vi "Build Per Cycle CO CO2 Array.vi"(4 "Burner ON":bool, 6 "Start Analyzing Cycles at":u16=14, 7 "Conditions":T8, 8 "error in":errorcluster, 11 "PLC Data In":T1 {"PLC Data - LDO"."Timing"."Absolute Time" format="%<%H:%M:%S%3u>t"; "PLC Data - LDO"."Timing"."Display Time" format="%#.20f"; "PLC Data - LDO"."Timing"."Test Time Ref" format="%#.20f"; "PLC Data - LDO"."Timing"."Precondition Time Ref" format="%#.20f"; "PLC Data - LDO"."Timing"."First Call Time Ref" format="%#.20f"; "PLC Data - FVIR"."Timing"."Absolute Time" format="%<%H:%M:%S%3u>t"; "PLC Data - FVIR"."Timing"."Display Time" format="%#.20f"; "PLC Data - FVIR"."Timing"."Test Time Ref" format="%#.20f"; "PLC Data - FVIR"."Timing"."Precondition Time Ref" format="%#.20f"; "PLC Data - FVIR"."Timing"."First Call Time Ref" format="%#.20f"}) -> (0 "error out":errorcluster, 3 "PLC Data Out":T1 {"PLC Data - LDO"."Timing"."Absolute Time" format="%<%H:%M:%S%3u>t"; "PLC Data - LDO"."Timing"."Display Time" format="%#.20f"; "PLC Data - LDO"."Timing"."Test Time Ref" format="%#.20f"; "PLC Data - LDO"."Timing"."Precondition Time Ref" format="%#.20f"; "PLC Data - LDO"."Timing"."First Call Time Ref" format="%#.20f"; "PLC Data - FVIR"."Timing"."Absolute Time" format="%<%H:%M:%S%3u>t"; "PLC Data - FVIR"."Timing"."Display Time" format="%#.20f"; "PLC Data - FVIR"."Timing"."Test Time Ref" format="%#.20f"; "PLC Data - FVIR"."Timing"."Precondition Time Ref" format="%#.20f"; "PLC Data - FVIR"."Timing"."First Call Time Ref" format="%#.20f"})   [LabVIEW 2020]
uses:
  Terminate Condition ENUM.ctl
  Modbus/Modbus PLC Data All.ctl
  Modbus/Modbus FVIR Control.ctl
  Modbus/Modbus Timing.ctl
  <vilib>/Utility/miscctls.llb/LVDateTimeRec.ctl
  Modbus/Modbus LDO Control.ctl
  WritingDataFile/Data to Save.ctl
  Terminate Conditions Cluster.ctl
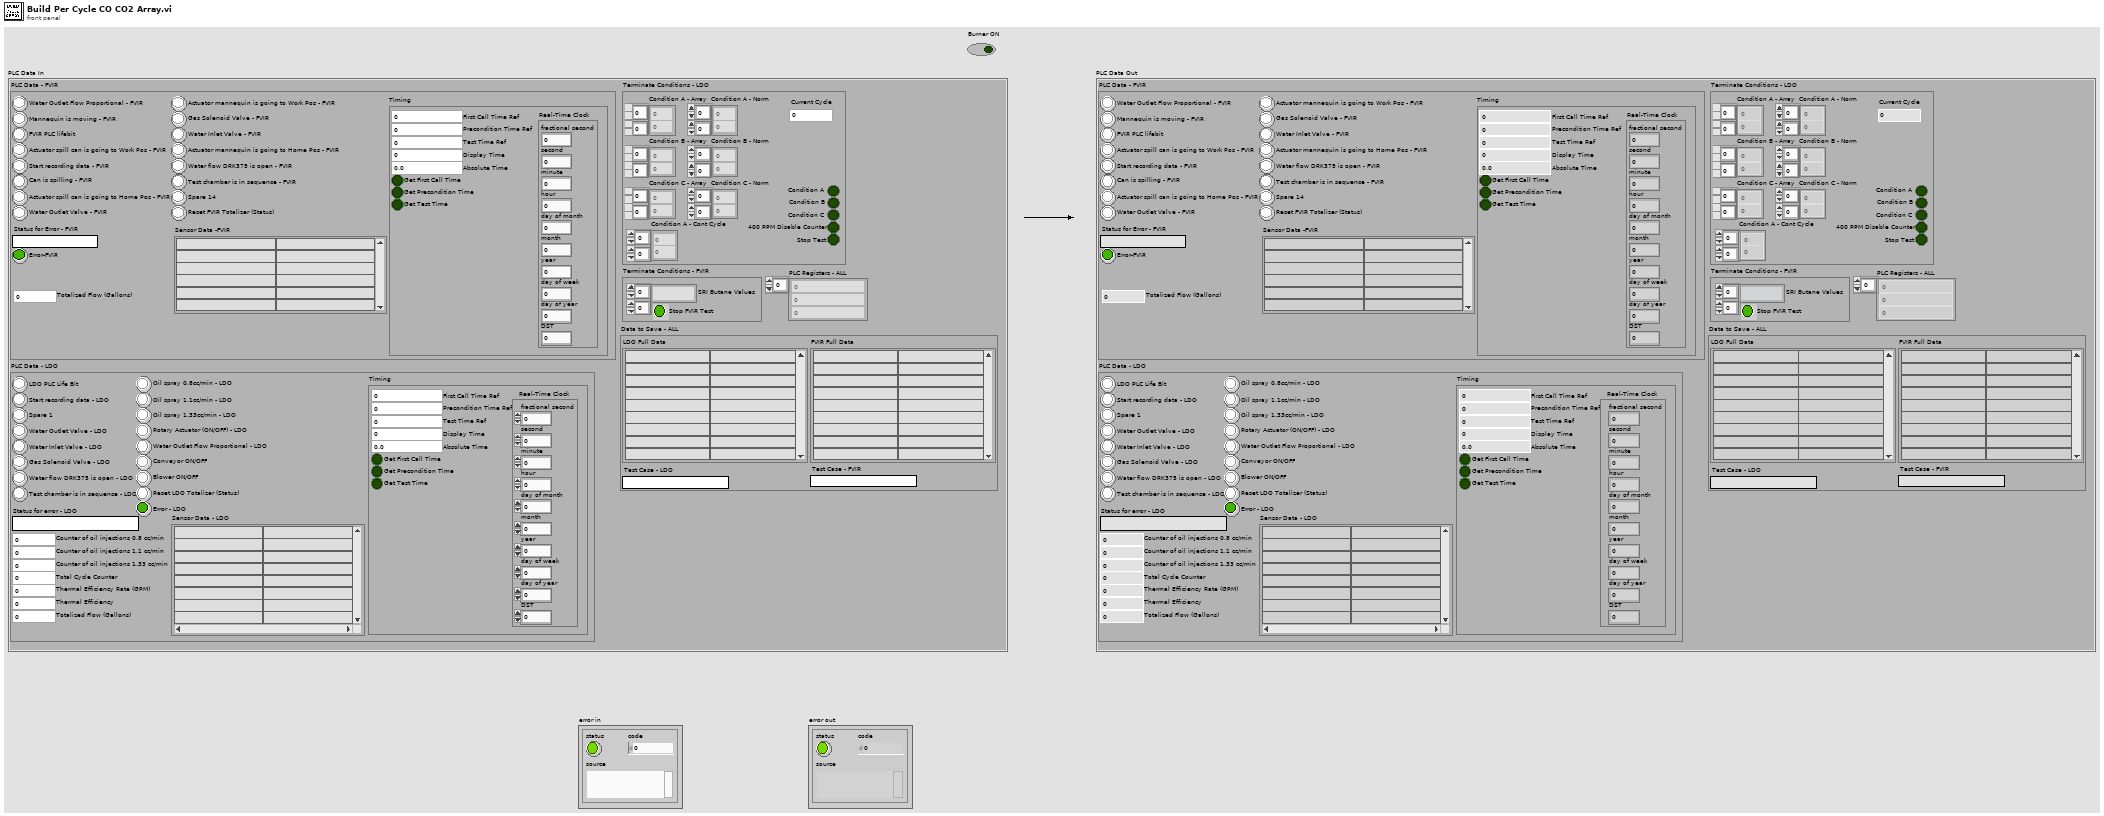
[diagram p1: front panel]
types:
  T1 = typedef "Modbus PLC Data All.ctl" = cluster{"PLC Data - FVIR":T2, "PLC Data - LDO":T5, "PLC Registers - ALL":i16[], "Data to Save - ALL":T6, "Terminate Conditions - LDO":T7, "Terminate Conditions - FVIR":cluster{"SRI Butane Values":string[][], "Stop FVIR Test":bool}}
  T2 = typedef "Modbus FVIR Control.ctl" = cluster{"Reset FVIR Totalizer (Status)":bool, "Spare 14":bool, "Actuator mannequin is going to Work Pos - FVIR":bool, "Actuator mannequin is going to Home Pos - FVIR":bool, "Test chamber is in sequence - FVIR ":bool, "Water flow DRK375 is open - FVIR":bool, "Gas Solenoid Valve - FVIR":bool, "Water Inlet Valve - FVIR":bool, "Water Outlet Flow Proportional - FVIR":bool, "Start recording data - FVIR":bool, "Actuator spill can is going to Work Pos - FVIR":bool, "Actuator spill can is going to Home Pos - FVIR":bool, "Water Outlet Valve - FVIR":bool, "Can is spilling - FVIR":bool, "Mannequin is moving - FVIR":bool, "FVIR PLC lifebit":bool, "Status for Error - FVIR":string, "Error-FVIR":bool, "Sensor Data -FVIR":string[][], "Totalized Flow (Gallons)":dbl, "Timing":T3}
  T3 = typedef "Modbus Timing.ctl" = cluster{"First Call Time Ref":dbl, "Precondition Time Ref":dbl, "Test Time Ref":dbl, "Get First Call Time":bool, "Get Precondition Time":bool, "Get Test Time":bool, "Display Time":dbl, "Real-Time Clock":T4, "Absolute Time":dbl}
  T4 = typedef "LVDateTimeRec.ctl" = cluster{"fractional second":dbl, "second":i32, "minute":i32, "hour":i32, "day of month":i32, "month":i32, "year":i32, "day of week":i32, "day of year":i32, "DST":i32}
  T5 = typedef "Modbus LDO Control.ctl" = cluster{"LDO PLC Life Bit":bool, "Start recording data - LDO":bool, "Spare 1":bool, "Water Outlet Valve - LDO":bool, "Water Inlet Valve - LDO":bool, "Gas Solenoid Valve - LDO":bool, "Water flow DRK375 is open - LDO":bool, "Test chamber is in sequence - LDO":bool, "Oil spray 0.8cc/min - LDO":bool, "Oil spray 1.1cc/min - LDO":bool, "Oil spray 1.33cc/min - LDO":bool, "Rotary Actuator (ON/OFF) - LDO":bool, "Water Outlet Flow Proportional - LDO":bool, "Conveyor ON/OFF":bool, "Blower ON/OFF":bool, "Reset LDO Totalizer (Status)":bool, "Status for error - LDO":string, "Error - LDO":bool, "Sensor Data - LDO":string[][], "Thermal Efficiency Rate (GPM)":dbl, "Thermal Efficiency":dbl, "Totalized Flow (Gallons)":dbl, "Counter of oil injections 1.33 cc/min":u16, "Total Cycle Counter":u16, "Counter of oil injections 1.1 cc/min":u16, "Counter of oil injections 0.8 cc/min":u16, "Timing":T3}
  T6 = typedef "Data to Save.ctl" = cluster{"LDO Full Data":string[][], "FVIR Full Data":string[][], "Test Case - FVIR":string, "Test Case - LDO":string}
  T7 = typedef "Terminate Conditions Cluster.ctl" = cluster{"Condition B - Array":dbl[][], "Current Cycle":u16, "Condition C - Array":dbl[][], "Condition A - Array":dbl[][], "400 PPM Disable Counter":bool, "Condition A - Norm":dbl[][], "Condition B - Norm":dbl[][], "Condition C - Norm":dbl[][], "Condition A":bool, "Condition B":bool, "Condition C":bool, "Condition A - Cont Cycle":dbl[][], "Stop Test":bool}
  T8 = typedef "Terminate Condition ENUM.ctl" = enum16{"Condition A", "Condition B", "Condition C"}
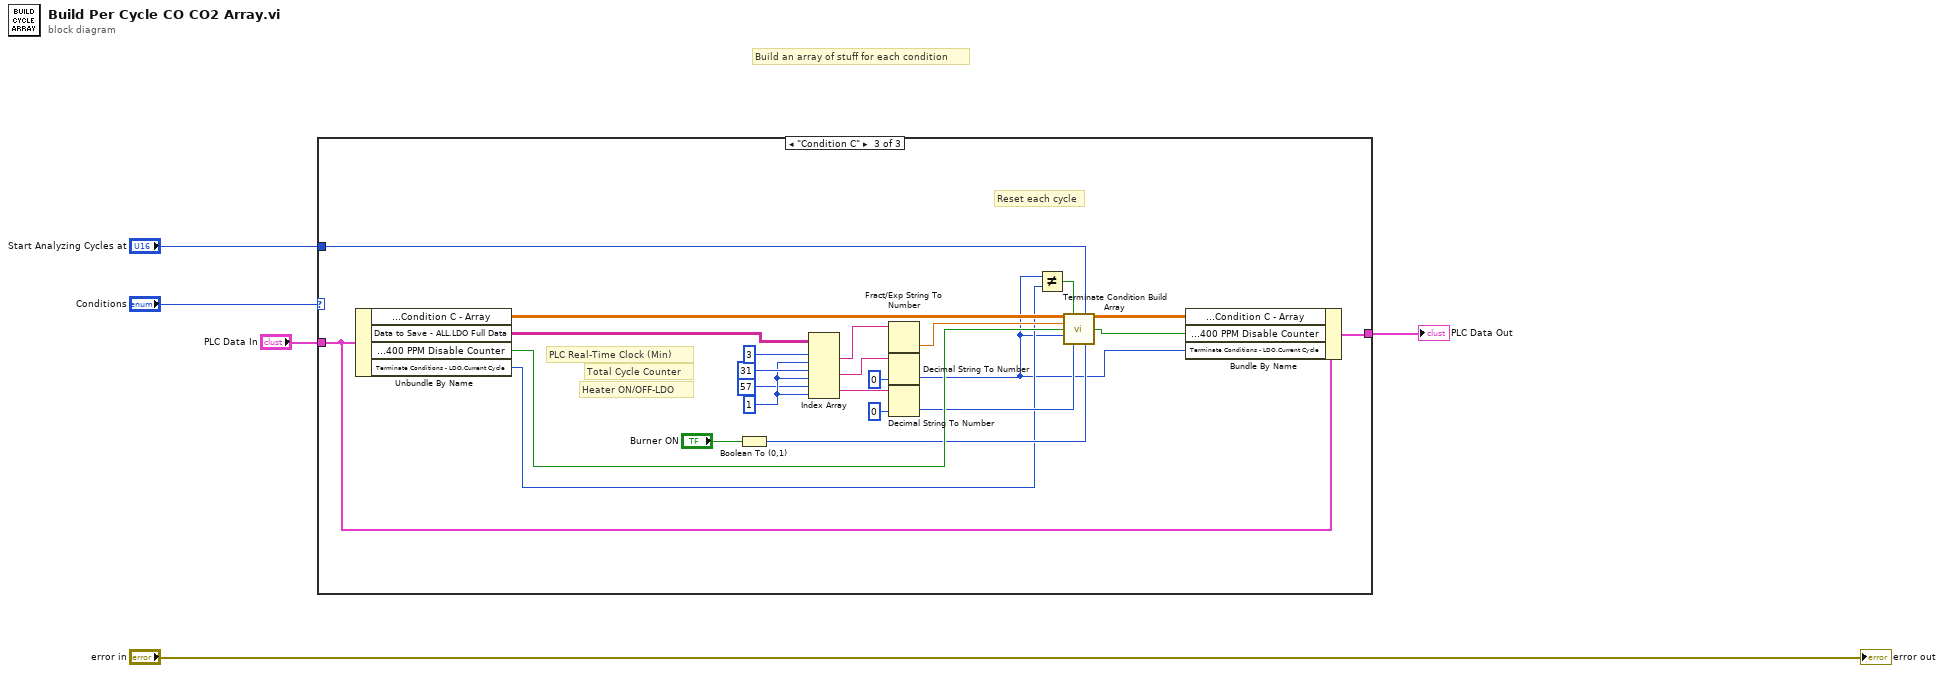
[diagram p0: block diagram]
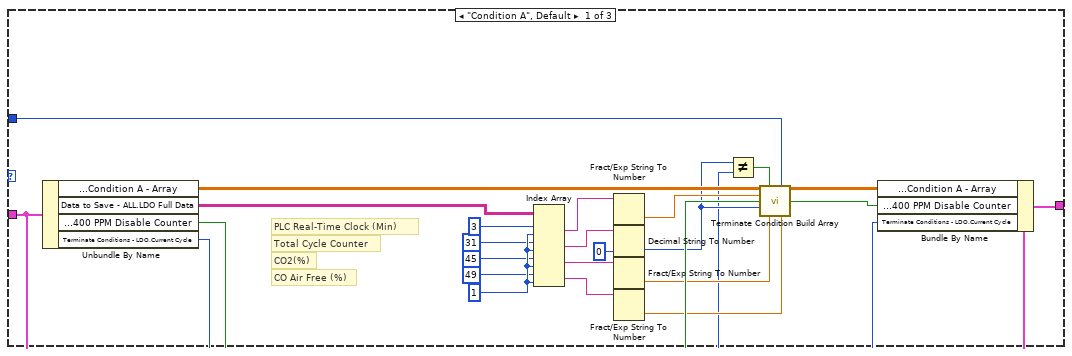
[diagram p2: hidden frame]
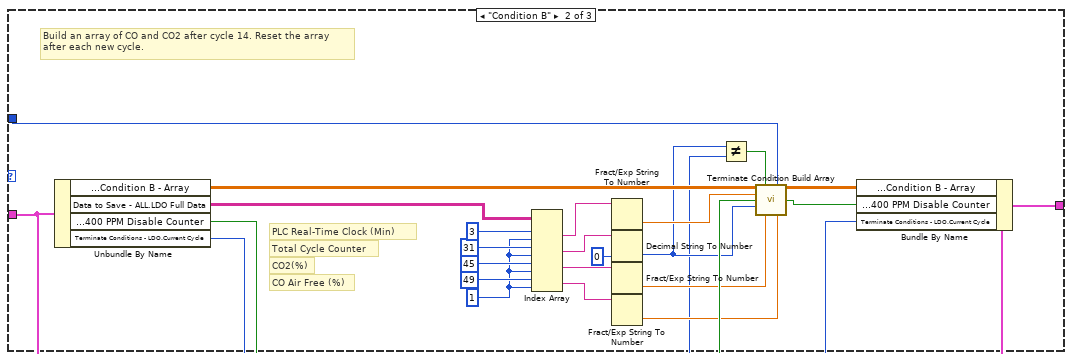
[diagram p3: hidden frame]
diagram:
  # "Build an array of stuff for each condition"
  n1 = case shown="\"Condition C\"" "Conditions" {
    tunnel: "PLC Data In" -> [w6 w42 w58]
    tunnel: "Start Analyzing Cycles at" -> [w16 w31 w59]
    tunnel: [w7 w41 w54] -> w1
    frame "Condition A", Default {
      w23 = 1 ("disabled index (col)")
      # "CO Air Free (%)"
      # "CO2(%)"
      # "Total Cycle Counter"
      # "PLC Real-Time Clock (Min)"
      n2 = Unbundle By Name(w6) -> ("Terminate Conditions - LDO.Condition A - Array"=w18:dbl[][], "Data to Save - ALL.LDO Full Data"=w19:string[][], "Terminate Conditions - LDO.400 PPM Disable Counter"=w15:bool, "Terminate Conditions - LDO.Current Cycle"=w9:u16)
      n3 = Index Array(array=w19, index (row) #1=3 ("disabled index (col)"), index (col) #1=w23, index (row) #2=31 ("index (col)"), index (col) #2=w23, index (row) #3=45 ("index (col)"), index (col) #3=w23, index (row) #4=49 ("index (col)"), index (col) #4=w23) -> (element #1=w26:string, element #2=w27:string, element #3=w28:string, element #4=w29:string)
      n4 = Fract/Exp String To Number(string=w26) -> (number=w14:dbl)  [unwired: 3 in, 1 out]
      n5 = Decimal String To Number(string=w27, default (0L)=u16 0 ("default (0 I32)")) -> (number=w10:u16)  [unwired: 1 in, 1 out]
      n6 = Fract/Exp String To Number(string=w28) -> (number=w13:dbl)  [unwired: 3 in, 1 out]
      n7 = Fract/Exp String To Number(string=w29) -> (number=w12:dbl)  [unwired: 3 in, 1 out]
      n8 = Not Equal?(x=w10, y=w9) -> (x != y?=w11:bool)
      n9 = call "Terminate Condition Build Array.vi"("Array in"=w18, "Reset Array?"=w11, "Start Analyzing Cycles at"=w16, "PLC Real-Time Clock (Min)"=w14, "Disable 400 PPM Counter In"=w15, "Total Cycle Counter"=w10, "Column 2"=w13, "Column 3"=w12) -> ("Array out"=w17:dbl[][], "Disable 400 PPM Counter Our"=w8:bool)  [unwired: 5 in, 1 out]
      n10 = Bundle By Name(cluster=w6, "Terminate Conditions - LDO.Condition A - Array"=w17, "Terminate Conditions - LDO.400 PPM Disable Counter"=w8, "Terminate Conditions - LDO.Current Cycle"=w9) -> (w7:T1)
    }
    frame "Condition B" {
      w49 = 1 ("disabled index (col)")
      # "Build an array of CO and CO2 after cycle 14. Reset the array\nafter each new cycle."
      # "CO Air Free (%)"
      # "CO2(%)"
      # "Total Cycle Counter"
      # "PLC Real-Time Clock (Min)"
      n11 = Unbundle By Name(w42) -> ("Terminate Conditions - LDO.Condition B - Array"=w40:dbl[][], "Data to Save - ALL.LDO Full Data"=w43:string[][], "Terminate Conditions - LDO.400 PPM Disable Counter"=w36:bool, "Terminate Conditions - LDO.Current Cycle"=w30:u16)
      n12 = Index Array(array=w43, index (row) #1=3 ("disabled index (col)"), index (col) #1=w49, index (row) #2=31 ("index (col)"), index (col) #2=w49, index (row) #3=45 ("index (col)"), index (col) #3=w49, index (row) #4=49 ("index (col)"), index (col) #4=w49) -> (element #1=w45:string, element #2=w46:string, element #3=w47:string, element #4=w48:string)
      n13 = Fract/Exp String To Number(string=w45) -> (number=w37:dbl)  [unwired: 3 in, 1 out]
      n14 = Decimal String To Number(string=w46, default (0L)=u16 0 ("default (0 I32)")) -> (number=w35:u16)  [unwired: 1 in, 1 out]
      n15 = Fract/Exp String To Number(string=w47) -> (number=w34:dbl)  [unwired: 3 in, 1 out]
      n16 = Fract/Exp String To Number(string=w48) -> (number=w33:dbl)  [unwired: 3 in, 1 out]
      n17 = Not Equal?(x=w35, y=w30) -> (x != y?=w38:bool)
      n18 = call "Terminate Condition Build Array.vi"("Array in"=w40, "Reset Array?"=w38, "Start Analyzing Cycles at"=w31, "PLC Real-Time Clock (Min)"=w37, "Disable 400 PPM Counter In"=w36, "Total Cycle Counter"=w35, "Column 2"=w34, "Column 3"=w33) -> ("Array out"=w39:dbl[][], "Disable 400 PPM Counter Our"=w32:bool)  [unwired: 5 in, 1 out]
      n19 = Bundle By Name(cluster=w42, "Terminate Conditions - LDO.Condition B - Array"=w39, "Terminate Conditions - LDO.400 PPM Disable Counter"=w32, "Terminate Conditions - LDO.Current Cycle"=w30) -> (w41:T1)
    }
    frame "Condition C" {
      w71 = 1 ("disabled index (col)")
      # "Reset each cycle"
      # "Heater ON/OFF-LDO"
      # "Total Cycle Counter"
      # "PLC Real-Time Clock (Min)"
      n20 = Unbundle By Name(w58) -> ("Terminate Conditions - LDO.Condition C - Array"=w66:dbl[][], "Data to Save - ALL.LDO Full Data"=w67:string[][], "Terminate Conditions - LDO.400 PPM Disable Counter"=w64:bool, "Terminate Conditions - LDO.Current Cycle"=w61:u16)
      n21 = Boolean To (0,1)(Boolean="Burner ON") -> (0, 1=w62:i16)
      n22 = Index Array(array=w67, index (row) #1=3 ("disabled index (col)"), index (col) #1=w71, index (row) #2=31 ("index (col)"), index (col) #2=w71, index (row) #3=57 ("index (col)"), index (col) #3=w71) -> (element #1=w76:string, element #2=w77:string, element #3=w68:string)
      n23 = Fract/Exp String To Number(string=w76) -> (number=w65:dbl)  [unwired: 3 in, 1 out]
      n24 = Decimal String To Number(string=w77, default (0L)=u16 0 ("default (0 I32)")) -> (number=w55:u16)  [unwired: 1 in, 1 out]
      n25 = Decimal String To Number(string=w68, default (0L)=u16 0 ("default (0 I32)")) -> (number=w63:u16)  [unwired: 1 in, 1 out]
      n26 = Not Equal?(x=w55, y=w61) -> (x != y?=w60:bool)
      n27 = call "Terminate Condition Build Array.vi"("Array in"=w66, "Reset Array?"=w60, "Start Analyzing Cycles at"=w59, "PLC Real-Time Clock (Min)"=w65, "Disable 400 PPM Counter In"=w64, "Total Cycle Counter"=w55, "Column 2"=w63, "Column 3"=w62) -> ("Array out"=w57:dbl[][], "Disable 400 PPM Counter Our"=w56:bool)  [unwired: 5 in, 1 out]
      n28 = Bundle By Name(cluster=w58, "Terminate Conditions - LDO.Condition C - Array"=w57, "Terminate Conditions - LDO.400 PPM Disable Counter"=w56, "Terminate Conditions - LDO.Current Cycle"=w55) -> (w54:T1)
    }
  }
  "PLC Data Out" <- w1
  "error out" <- "error in"
